vi "DrawField.vi"(7 "ForceDraw?":bool, 8 "error in (no error)":errorcluster, 11 "Pong in":refnum<class "Pong.lvclass">) -> (0 "error out":errorcluster, 3 "Pong out":refnum<class "Pong.lvclass">)   [LabVIEW 2019, in "RT_Game.lvlib" / "Pong.lvclass"]
uses:
  Pong.lvclass
  C:/Users/FreshBob/Dropbox/VIs/myRIO_GameConsole/RT/RT_Game/Game/Game.lvclass
  Game/Game.lvclass/Game.ctl
  Game/Coordinate.ctl
  Game/Read Player1Score.vi
  Game/Read Player2Score.vi
  Game/Game.lvclass
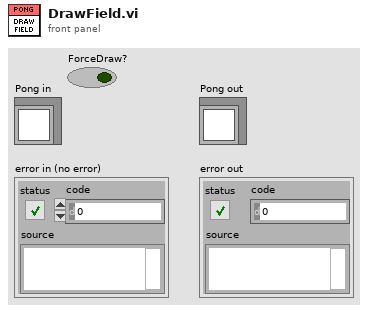
[diagram p1: front panel]
types:
  T1 = typedef "RT_Game.lvlib/Game.lvclass/Coordinate.ctl" = cluster{"x":dbl, "y":dbl}
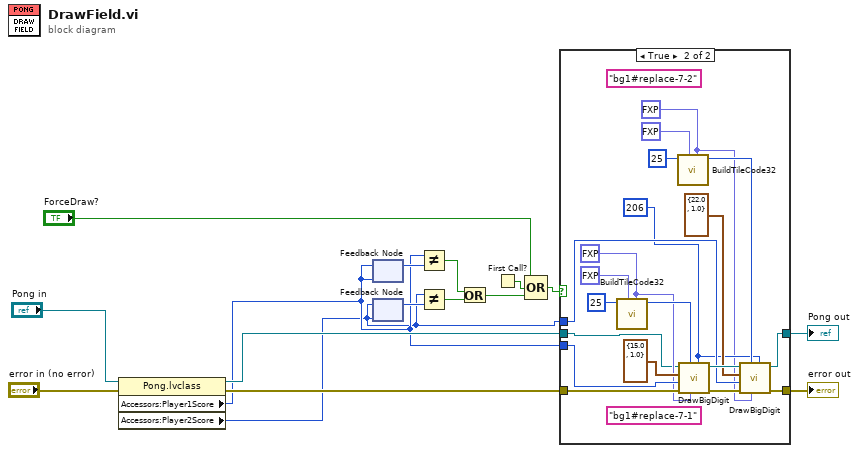
[diagram p0: block diagram]
diagram:
  n1 = property class="Pong.lvclass"(reference="Pong in", error in="error in (no error)") -> (reference out=w3:refnum<class "Pong.lvclass">, error out=w5:errorcluster, "Accessors:Player1Score"=w2:i32, "Accessors:Player2Score"=w1:i32)
  n2 = feedback-in #1(w2) -> ()
  n3 = feedback #1(w2) -> (w13:i32)
  n4 = feedback #2(w1) -> (w12:i32)
  n5 = feedback-in #2(w1) -> ()
  n6 = Not Equal?(x=w2, y=w13) -> (x != y?=w11:bool)
  n7 = Not Equal?(x=w1, y=w12) -> (x != y?=w10:bool)
  n8 = Or(x=w11, y=w10) -> (x .or. y?=w9:bool)
  n9 = First Call?() -> (First Call?: T/F=w7:bool)
  n10 = Compound Arithmetic op=OR("ForceDraw?", w7, w9) -> (w8:bool)
  n11 = case shown="True" w8 {
    tunnel: [w17 w37] -> w16
    tunnel: [w18 w36] -> w15
    tunnel: w2 -> [_ w31]
    tunnel: w1 -> [_ w30]
    tunnel: w5 -> [w17 w22]
    tunnel: w3 -> [w18 w19]
    frame False {
    }
    frame True {
      w23 = u32 206
      w20 = fxp<+,3,3> 2.0 ("replacecolor")
      w21 = fxp<+,3,3> 1.0 ("replacecolor")
      (unwired) "bg1#replace-7-2" ("LetterTile")
      (unwired) "bg1#replace-7-1" ("LetterTile")
      n12 = call "BuildTileCode32.vi"("replacecolor"=w21, "color_to_replace"=fxp<+,3,3> 7.0, "Tilenumber"=u32 25) -> ("TileCode"=w24:u32)  [unwired: 8 in]
      n13 = call "BuildTileCode32.vi"("replacecolor"=w20, "color_to_replace"=fxp<+,3,3> 7.0, "Tilenumber"=u32 25) -> ("TileCode"=w25:u32)  [unwired: 8 in]
      n14 = call "DrawBigDigit.vi"("BgTile"=w23, "color"=w21, "LetterTile"=w24, "error in (no error)"=w22, "Digit"=w31, "Position"=T1 {"x"=15.0, "y"=1.0} ("position"), "Game in"=w19) -> ("error out"=w34:errorcluster, "Game out"=w35:refnum<class "Pong.lvclass">)  [unwired: 3 in]
      n15 = call "DrawBigDigit.vi"("BgTile"=w23, "color"=w20, "LetterTile"=w25, "error in (no error)"=w34, "Digit"=w30, "Position"=T1 {"x"=22.0, "y"=1.0} ("position"), "Game in"=w35) -> ("error out"=w37:errorcluster, "Game out"=w36:refnum<class "Pong.lvclass">)  [unwired: 3 in]
    }
  }
  "error out" <- w16
  "Pong out" <- w15
